vi "vr-main-ctl.vi"() -> ()   [LabVIEW 2013]
panel:
  in  "停止按钮":bool
  in  "angle 2":i16(slide) scale=-45.0..180.0
  in  "angle":i16(slide) scale=0.0..150.0
  out "三维图片":refnum<vi>(3d-picture)
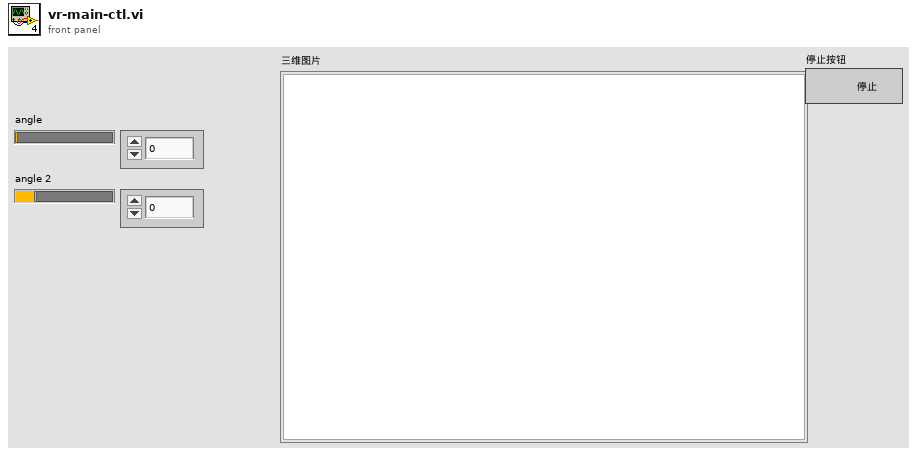
[diagram p1: front panel]
types:
  T1 = cluster{"zuoqian1":refnum<vi>, "zuoqian2":refnum<vi>, "zuoqian3":refnum<vi>}
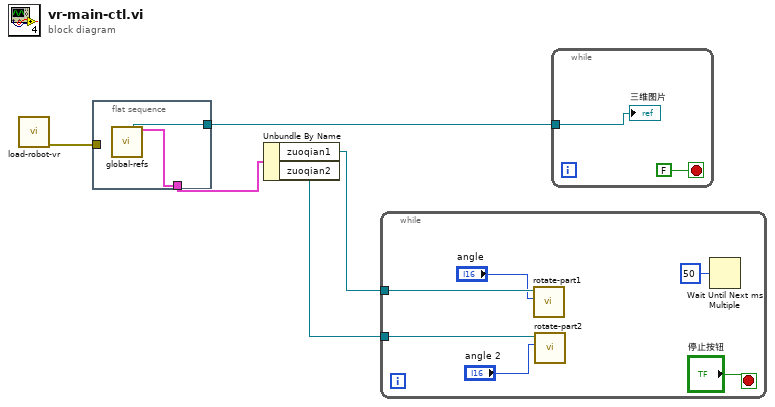
[diagram p0: block diagram]
diagram:
  n1 = call "load-robot-vr.vi"() -> ("错误输出"=w5:errorcluster)  [unwired: 11 in]
  n2 = flat-sequence {
    tunnel: [w7] -> w1
    tunnel: [w6] -> _
    tunnel: w5 -> [_]
    tunnel: [w6] -> w4
    frame #0 {
      n3 = call "global-refs.vi"() -> ("RobotRef"=w7:refnum<vi>, "ZuoQianRef"=w6:T1)  [unwired: 10 in, 4 out]
    }
  }
  n4 = Unbundle By Name(w4) -> ("zuoqian1"=w3:refnum<vi>, "zuoqian2"=w2:refnum<vi>)
  n5 = while {
    tunnel: w3 -> [w13]
    tunnel: w2 -> [w12]
    stop <- "停止按钮" stop-if-true
    n6 = call "rotate-part1.vi"("Angle"="angle", "SceneObject输入"=w13) -> ()  [unwired: 8 in, 2 out]
    n7 = call "rotate-part2.vi"("Angle"="angle 2", "SceneObject输入"=w12) -> ()  [unwired: 8 in, 2 out]
    n8 = Wait Until Next ms Multiple(millisecond multiple=u32 50 ("毫秒倍数")) -> ()  [unwired: 1 out]
  }
  n9 = while {
    tunnel: w1 -> [w15]
    stop <- FALSE stop-if-true
    "三维图片" <- w15
  }
